vi "Magazine_Execute.vi"() -> ()   [LabVIEW 2020]
uses:
  Globals/Magazine_Globals.vi
  Globals/Sensor_Values.vi
panel:
  in  "Kd":dbl
  in  "Ki":dbl
  in  "Kp":dbl
  in  "Earlnator":dbl
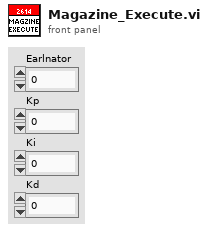
[diagram p1: front panel]
types:
  T1 = typedef "Magazine_Cluster.ctl" = cluster{"Control_States":T2, "Manual_Magazine":dbl, "Auto_Magazine":bool}
  T2 = typedef "Magazine_Control_States.ctl" = enum16{"No-Op", "Manual_Control", "Load", "Firing"}
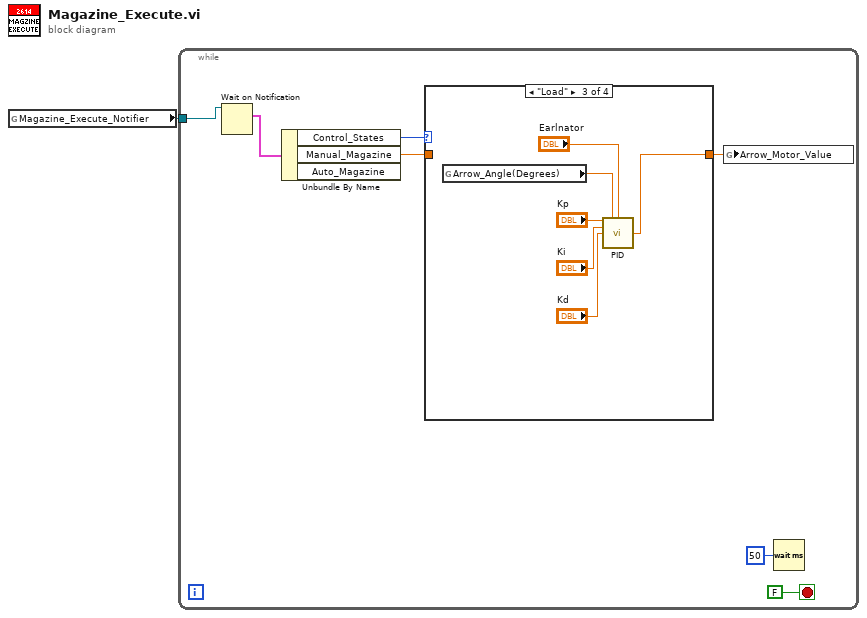
[diagram p0: block diagram]
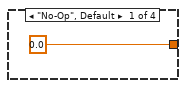
[diagram p2: hidden frame]
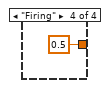
[diagram p4: hidden frame]
diagram:
  n1 = global read "Magazine_Globals.vi" "Magazine_Execute_Notifier"() -> (w1:refnum<notifier>)
  n2 = while {
    tunnel: w1 -> [w8]
    stop <- FALSE stop-if-true
    n3 = Wait on Notification(notifier=w8) -> (notification=w5:T1)  [unwired: 3 in, 3 out]
    n4 = Unbundle By Name(w5) -> ("Control_States"=w4:T2, "Manual_Magazine"=w3:dbl)  [unwired: 1 out]
    n5 = case shown="\"Load\"" w4 {
      tunnel: [0.0 w10 w11 0.5 ("Command")] -> w2
      tunnel: w3 -> [_ w10 _ _]
      frame "No-Op", Default {
      }
      frame "Manual_Control" {
      }
      frame "Load" {
        n6 = global read "Sensor_Values.vi" "Arrow_Angle(Degrees)"() -> (w15:dbl)
        n7 = call "PID.vi"("Kp"="Kp", "Process Variable"=w15, "Goal"="Earlnator", "Ki"="Ki", "Kd"="Kd") -> ("Command"=w11:dbl)  [unwired: 8 in, 2 out]
      }
      frame "Firing" {
      }
    }
    n8 = global write "Magazine_Globals.vi" "Arrow_Motor_Value"(w2) -> ()
    n9 = Wait (ms)(milliseconds to wait=u32 50) -> ()  [unwired: 1 out]
  }
